vi "Scalar_Data_3.vi"() -> ()   [LabVIEW 2012]
panel:
  out "Scalar Data 3":u16[](array[numeric])
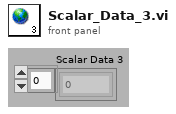
[diagram p1: front panel]
diagram:
